vi "Read Tag Description.vi"(8 "error in (no error)":errorcluster, 11 "Tag Name":string) -> (0 "error out":errorcluster, 3 "Description":string)   [LabVIEW 2010, in "Current Value Table.lvlib"]
doc: "This VI will retrieve the description of a single tag. It can be easily modified to retrieve descriptions for a group of tags."
uses:
  Current Value Table.lvlib
  FGVs/Tag Memory Methods.ctl
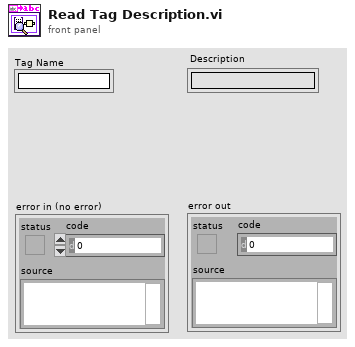
[diagram p1: front panel]
types:
  T1 = typedef "Current Value Table.lvlib/Tag Memory Methods.ctl" = enum16{"Clear", "Read Tag Index", "Read Tag Indices", "Generate Group", "Add Tag", "Overwrite Tag", "Read Description", "Get Stored Tags"}
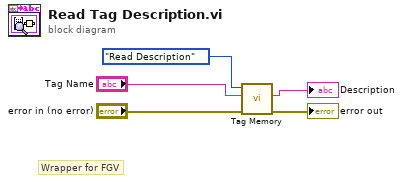
[diagram p0: block diagram]
diagram:
  # "Wrapper for FGV"
  n1 = call "Tag Memory.vi"("error in (no error)"="error in (no error)", "Tag"="Tag Name", "Method"=Tag_Memory_Methods."Read Description") -> ("error out"=→"error out":errorcluster, "Description"=→"Description":string)  [unwired: 3 in, 4 out]
